vi "Part 2.vi"(11 "Input":string) -> (3 "Output":i64)   [LabVIEW 2021]
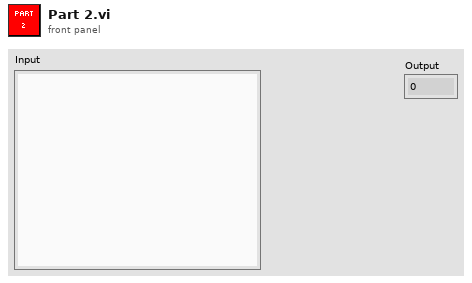
[diagram p1: front panel]
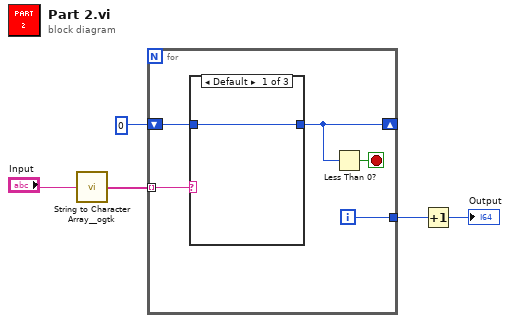
[diagram p0: block diagram]
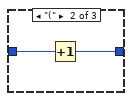
[diagram p2: hidden frame]
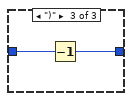
[diagram p3: hidden frame]
diagram:
  n1 = call <userlib>:"String to Character Array__ogtk.vi"("Input String"="Input") -> ("Character Array"=w4:string[])
  n2 = for {
    tunnel: w4 -> [w10] mode=indexing
    shift-right: [w7] -> _
    shift-left: 0 -> [w9]
    tunnel: [w6] -> w2
    i -> [w6]
    stop <- w8 stop-if-true
    n3 = case shown="Default" w10 {
      tunnel: w9 -> [w11 w13 w15]
      tunnel: [w11 w12 w14] -> w7
      frame Default {
      }
      frame "(" {
        n4 = Increment(x=w13) -> (x+1=w12:i32)
      }
      frame ")" {
        n5 = Decrement(x=w15) -> (x-1=w14:i32)
      }
    }
    n6 = Less Than 0?(x=w7) -> (x < 0?=w8:bool)
  }
  n7 = Increment(x=w2) -> (x+1=→"Output":i32)
